vi "Test AI.vi"() -> ()   [LabVIEW 2023, in "AI.lvlib"]
uses:
  AI.lvlib
  Test Values.ctl
panel:
  out "PWM":T1
  out "B":T1
  out "A":T1
  out "Waveform Graph":waveform(dbl)[](graph)
  out "data":waveform(dbl)[](array[waveform])
  in  "timeout":dbl=10.0 format="%0.2f"
  in  "number of samples per channel":i32=-1
  out "error out":errorcluster
  in  "error in":errorcluster
  in  "Channel":string="ai0"
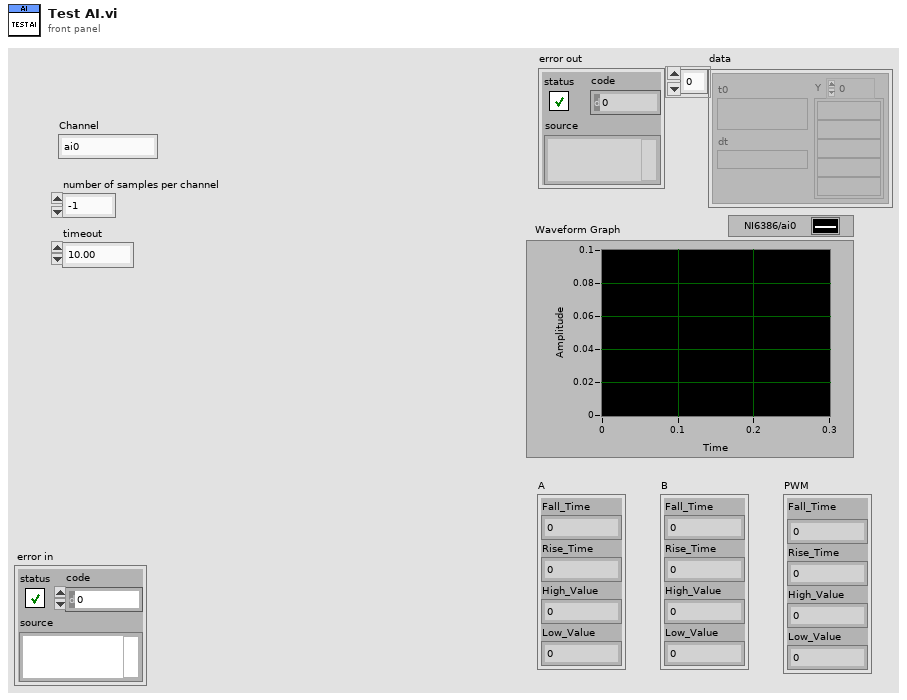
[diagram p1: front panel]
types:
  T1 = typedef "AI.lvlib/Test Values.ctl" = cluster{"Fall_Time":dbl, "Rise_Time":dbl, "High_Value":dbl, "Low_Value":dbl}
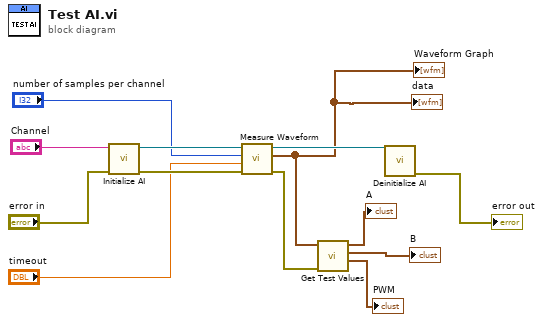
[diagram p0: block diagram]
diagram:
  n1 = call "Initialize AI.vi"("error in"="error in", "Channel"="Channel") -> ("error out"=w11:errorcluster, "task out"=w8:refnum<k21>)  [unwired: 8 in]
  n2 = call "Measure Waveform.vi"("task/channel"=w8, "error in"=w11, "timeout[s]"="timeout", "number of samples per channel"="number of samples per channel") -> ("error out"=w1:errorcluster, "data"=w5:waveform(dbl)[], "task out"=w10:refnum<k21>)  [unwired: 5 in]
  "data" <- w5
  "Waveform Graph" <- w5
  n3 = call "Get Test Values.vi"("error in"=w1, "Measurements"=w5) -> ("PWM"=→"PWM":T1, "B"=→"B":T1, "A"=→"A":T1)  [unwired: 6 in, 1 out]
  n4 = call "Deinitialize AI.vi"("task in"=w10) -> ("error out"=→"error out":errorcluster)  [unwired: 10 in]
